vi "Populate_Do.vi"(8 "error in (no error)":errorcluster, 9 "Value":string, 10 "Lower case name":string, 11 "Project Action Interface in":refnum<class "Project Action Interface.lvclass">) -> (0 "error out":errorcluster, 1 "Success?":bool, 3 "Project Action Interface out":refnum<class "Project Action Interface.lvclass">)   [LabVIEW 2020, in "ProjectBuilder.lvlib" / "Project Action Interface.lvclass"]
uses:
  Project Action Interface.lvclass
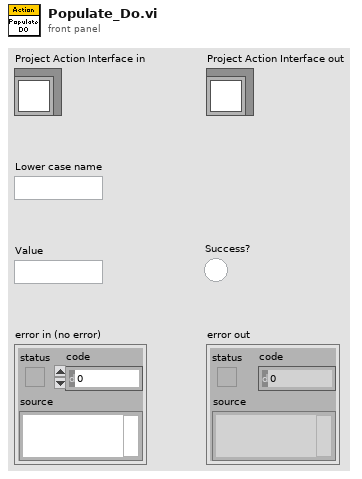
[diagram p1: front panel]
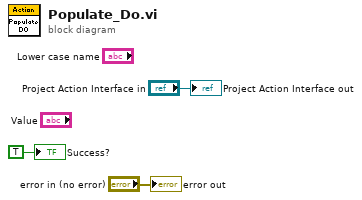
[diagram p0: block diagram]
diagram:
  "error out" <- "error in (no error)"
  "Project Action Interface out" <- "Project Action Interface in"
  "Success?" <- TRUE
